vi "test_DuplicateClientNames_CheckClientNameIsNotRepeated_NameInvalid.vi"() -> (6 "pass":bool, 8 "result":string, 15 "error out":errorcluster)   [LabVIEW 2021, in "MeasurementGenerator Tests.lvlib"]
uses:
  MeasurementGenerator Tests.lvlib
  <vilib>/ErrorRing/Error Ring.xnode
  Generator/_MeasurementClient Utility/MeasurementClient Editor.lvlib
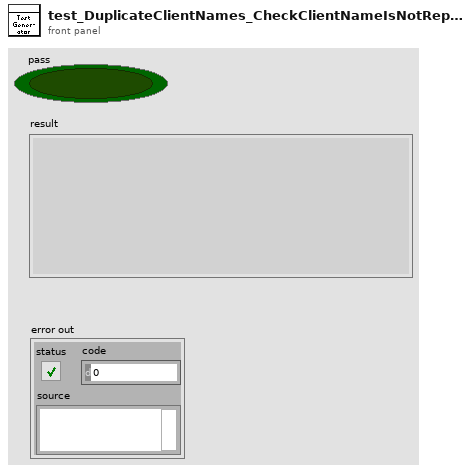
[diagram p1: front panel]
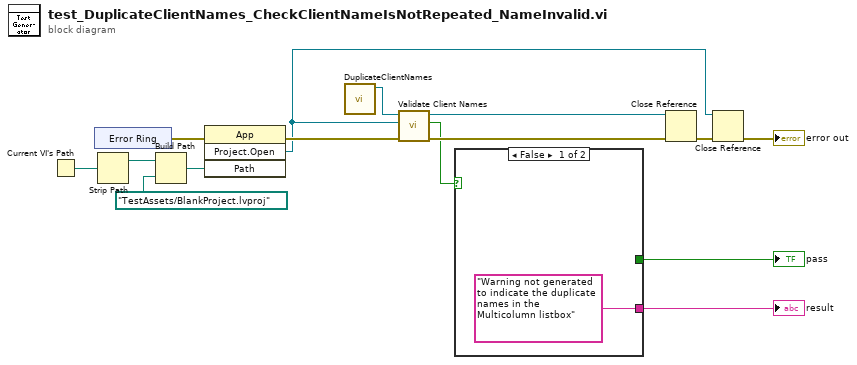
[diagram p0: block diagram]
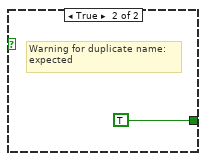
[diagram p2: hidden frame]
diagram:
  n1 = Current VI's Path() -> (path=w15:path)
  n2 = xnode "Error Ring"() -> ("error out"=w12:errorcluster)
  n3 = Strip Path(path=w15) -> (stripped path=w14:path)  [unwired: 1 out]
  n4 = Build Path(base path=w14, name or relative path=path "TestAssets/BlankProject.lvproj" ("path")) -> (appended path=w11:path)
  n5 = invoke class="App" method="Project.Open"(error in=w12, "Path"=w11) -> (error out=w8:errorcluster, "Project:Open"=w2:refnum<vi>)  [unwired: 2 in, 2 out]
  n6 = call "DuplicateClientNames.vi"() -> ("Multicolumn Listbox ref"=w6:refnum<vi>)  [unwired: 11 in]
  n7 = call "Validate Client Names.vi"("error in (no error)"=w8, "project ref"=w2, "multicolumnListbox in"=w6) -> ("error out"=w10:errorcluster, "warning?"=w7:bool, "multicolumnListbox out"=w4:refnum<vi>)  [unwired: 6 in]
  n8 = case shown="False" w7 {
    tunnel: ["Warning not generated to indicate the duplicate names in the Multicolumn listbox" ("format string") _] -> w1
    tunnel: [_ TRUE] -> w5
    frame False {
    }
    frame True {
      # "Warning for duplicate name:\nexpected"
    }
  }
  "pass" <- w5
  "result" <- w1
  n9 = Close Reference(reference=w4, error in (no error)=w10) -> (error out=w9:errorcluster)
  n10 = Close Reference(reference=w2, error in (no error)=w9) -> (error out=→"error out":errorcluster)
